vi "Create Unflatten Cases.vi"(4 "Fields":T1[](array[typedef]), 7 "Unflatten Refs":T4, 8 "error in (no error)":errorcluster, 11 "LV-Protoc in":refnum<class "LV-Protoc.lvclass">) -> (0 "error out":errorcluster, 1 "Bundlers":refnum<vi>[](array[refnum]), 2 "Decodes":refnum<vi>[](array[refnum]), 3 "LV-Protoc out":refnum<class "LV-Protoc.lvclass">)   [LabVIEW 2020, in "LV-Protoc.lvlib" / "LV-Protoc.lvclass"]
uses:
  LV-Protoc.lvclass
  Unflatten Refs.ctl
  LV-Proto/Field.ctl
  LV-Proto/Type.ctl
  LV-Proto/Proto Type.ctl
  <vilib>/Utility/traverseref.llb/TRef TravTarget.ctl
  Unflatten Template Case.ctl
  <vilib>/Utility/traverseref.llb/VI Scripting - Traverse.lvlib
  LV-Protoc.lvlib
  LV-Proto/LV-Proto.lvlib
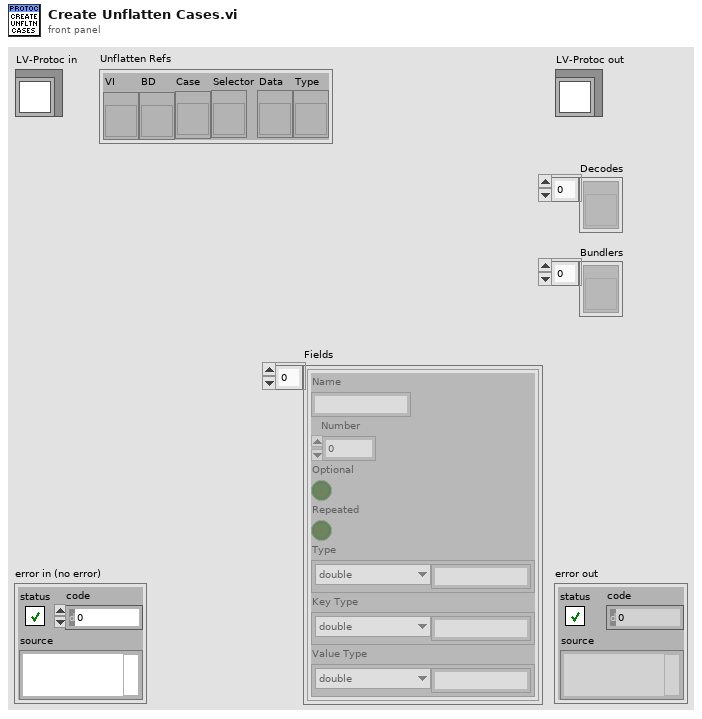
[diagram p1: front panel]
types:
  T1 = typedef "LV-Proto.lvlib/Field.ctl" = cluster{"Name":string, "Number":u32, "Optional":bool, "Repeated":bool, "Type":T2, "Key Type":T2, "Value Type":T2}
  T2 = typedef "LV-Proto.lvlib/Type.ctl" = cluster{"Type":T3, "Subtype":string}
  T3 = typedef "LV-Proto.lvlib/Proto Type.ctl" = enum16{"UNKNOWN", "double", "float", "int32", "int64", "uint32", "uint64", "sint32", "sint64", "fixed32", "fixed64", "sfixed32", "sfixed64", "bool", "string", "bytes", "enum", "map", "message"}
  T4 = typedef "LV-Protoc.lvlib/Unflatten Refs.ctl" = cluster{"VI":refnum<vi>, "BD":refnum<vi>, "Case":refnum<vi>, "Selector":refnum<vi>, "Data":refnum<vi>, "Type":refnum<vi>}
  T5 = typedef "LV-Protoc.lvlib/Unflatten Template Case.ctl" = enum16{"Unknown", "Scalar", "Array"}
  T6 = typedef "TRef TravTarget.ctl" = enum16{"FP", "BD", "Other"}
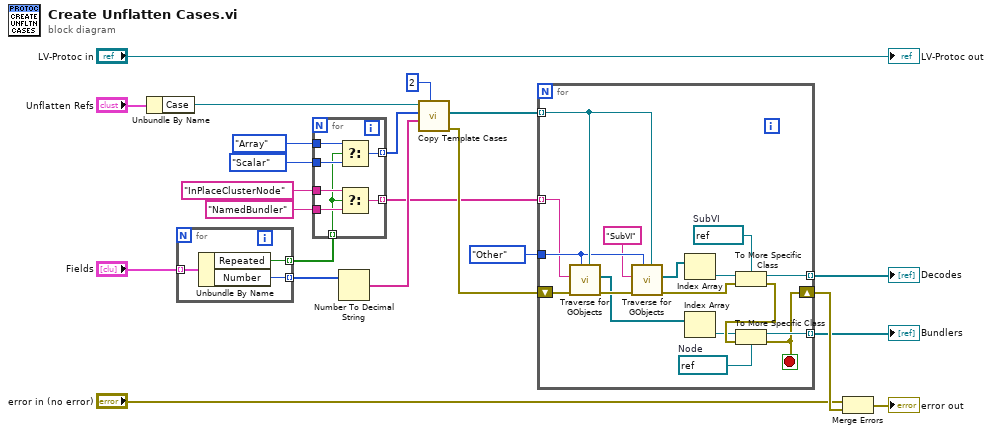
[diagram p0: block diagram]
diagram:
  n1 = Unbundle By Name("Unflatten Refs") -> ("Case"=w9:refnum<vi>)
  n2 = for {
    tunnel: "Fields" -> [w25] mode=indexing
    tunnel: [w24] -> w19 mode=indexing
    tunnel: [w23] -> w12 mode=indexing
    n3 = Unbundle By Name(w25) -> ("Repeated"=w23:bool, "Number"=w24:u32)
  }
  n4 = for {
    tunnel: w12 -> [w27] mode=indexing
    tunnel: Unflatten_Template_Case."Array" ("Unflatten Template Case") -> [w32]
    tunnel: Unflatten_Template_Case."Scalar" ("Unflatten Template Case") -> [w31]
    tunnel: [w30] -> w8 mode=indexing
    tunnel: "NamedBundler" -> [w29]
    tunnel: "InPlaceClusterNode" -> [w28]
    tunnel: [w26] -> w1 mode=indexing
    n5 = Select(t=w32, s=w27, f=w31) -> (s? t:f=w30:T5)
    n6 = Select(t=w28, s=w27, f=w29) -> (s? t:f=w26:string)
  }
  n7 = Number To Decimal String(number=w19) -> (decimal integer string=w7:string[])  [unwired: 1 in]
  n8 = call "Copy Template Cases.vi"("Template Case Count"=2, "Names"=w7, "Source Templates"=w8, "Case"=w9) -> ("error out"=w5:errorcluster, "Frames"=w4:refnum<vi>[])  [unwired: 6 in]
  n9 = for {
    tunnel: w4 -> [w46] mode=indexing
    shift-right: [w33] -> w22
    shift-left: w5 -> [w47]
    tunnel: TRef_TravTarget."Other" ("Traverse Target") -> [w45]
    tunnel: [w38] -> w14 mode=indexing
    tunnel: [w37] -> w13 mode=indexing
    tunnel: w1 -> [w34] mode=indexing
    stop <- w33 stop-if-true
    w36 = refnum<vi> refnum  # Node
    w39 = refnum<vi> refnum  # SubVI
    n10 = call <vilib>:"Traverse for GObjects.vi"("Other Refnum"=w46, "Traverse Target"=w45, "error in (no error)"=w47, "Class Name"=w34) -> ("error out"=w44:errorcluster, "References"=w43:refnum<vi>[])  [unwired: 4 in, 2 out]
    n11 = call <vilib>:"Traverse for GObjects.vi"("Other Refnum"=w46, "Traverse Target"=w45, "error in (no error)"=w44, "Class Name"="SubVI") -> ("error out"=w48:errorcluster, "References"=w42:refnum<vi>[])  [unwired: 4 in, 2 out]
    n12 = Index Array(array=w42) -> (element=w41:refnum<vi>)  [unwired: 1 in]
    n13 = Index Array(array=w43) -> (element=w40:refnum<vi>)  [unwired: 1 in]
    n14 = To More Specific Class(target class=w39, reference=w41, error in=w48) -> (specific class reference=w38:refnum<vi>, error out=w49:errorcluster)
    n15 = To More Specific Class(target class=w36, reference=w40, error in=w49) -> (specific class reference=w37:refnum<vi>, error out=w33:errorcluster)
  }
  "Decodes" <- w14
  "Bundlers" <- w13
  n16 = Merge Errors("error in (no error)", w22) -> (→"error out":errorcluster)
  "LV-Protoc out" <- "LV-Protoc in"
